vi "NI-DAQmxOLD.vi"() -> (0 "error out":errorcluster)   [LabVIEW 2022 SP3]
uses:
  Globals/Meas_global.vi
  <resource>/objmgr/daqmx.rc
  <vilib>/DAQmx/read.llb/DAQmx Read (Analog 2D DBL NChan NSamp).vi
  Sub_vis/Upload Data.ctl
  PWA/PWAtasksGLOBAL.vi
  <vilib>/DAQmx/create/channels.llb/DAQmx Create Channel (AI-Voltage-Basic).vi
  <vilib>/DAQmx/configure/timing.llb/DAQmx Timing (Sample Clock).vi
panel:
  out "FsReq":dbl
  out "FsRead":dbl format="%#_11g"
  out "input terminal configuration":i32(ring)=10106 items=["default"=-1, "RSE"=10083, "NRSE"=10078, "Differential"=10106, "Pseudodifferential"=12529]
  out "TotalSampPerChanAcquired":dbl=1024.0
  out "AvailSampPerChan":u32
  out "CurrReadPos":dbl=1024.0
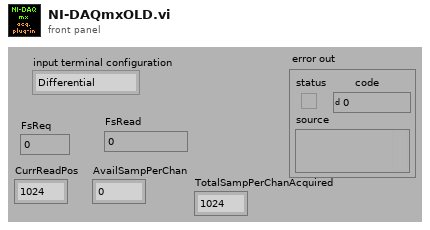
[diagram p1: front panel]
types:
  T1 = typedef "Analysis_info_cluster.ctl" = cluster{"Colour":u32, "Inst type":T2, "Inst name":string, "Symbol":string, "Code name":string, "Extra Info":string, "Inst Array":T3, "U":dbl, "u^2":dbl, "u^3":dbl, "u^4":dbl, "Skew_u":dbl, "Kurt_u":dbl, "Sd Error in Mean":dbl, "% u'/U":dbl, "X":dbl, "Y":dbl, "Z":dbl, "Timescale integral Estimate":dbl, "Sd Error in Variance":dbl, "Calib File":path, "Calib Constants":dbl[], "Output Position":bool, "Stats":enum16{"None", "Basic", "Full"}, "Av Sampling Rate":dbl, "Av No of Samples":dbl, "Total Meas Time (s)":dbl, "OrigChName":string, "Max value":dbl, "Min value":dbl, "Req Sample Rate Hz":dbl, "Sync Delay Time (s)":dbl, "Ch No":i16, "Device":string, "Use Latest Calib":bool, "Port":string, "Metadata Ch Names":string[], "Metadata Ch Values":string[], "Label":string, "chState":T4, "Point Drift":dbl, "inputConfig":string}
  T2 = typedef "Inst_type.ctl" = enum16{"Raw voltage", "Raw with zero offsetting", "Propeller anemometer", "Pressure Transducer", "Pitot-static tube", "Hot wire", "Cross wire 1", "Cross wire 2", "Generic Linear", "Generic Polynomial", "Generic BackPoly", "Fast FID", "Thermocouple", "Cold wire", "Pulsed Wire", "LDA Vel", "LDA Tran time", "LDA Arr time", "Microphone"}
  T3 = typedef "Instrument_Array.ctl" = enum16{"PWA", "LDA", "Analogue"}
  T4 = typedef "channelState.ctl" = enum32{"No Selection", "Solo", "Mute"}
  T5 = typedef "Device ID port info.ctl" = cluster{"Ch No":i16[], "Req Sampling Rate":dbl[], "Port":string, "Index":i32[]}
  T6 = typedef "Upload Data.ctl" = enum16{"Voltage Array", "Time Trace Cluster"}
  T7 = typedef "Setup.ctl" = enum16{"Run Program", "Show Setup", "Save Current Setup", "Setup Front Panel"}
  T8 = typedef "Rendezvous RefNum" = refnum<k1>
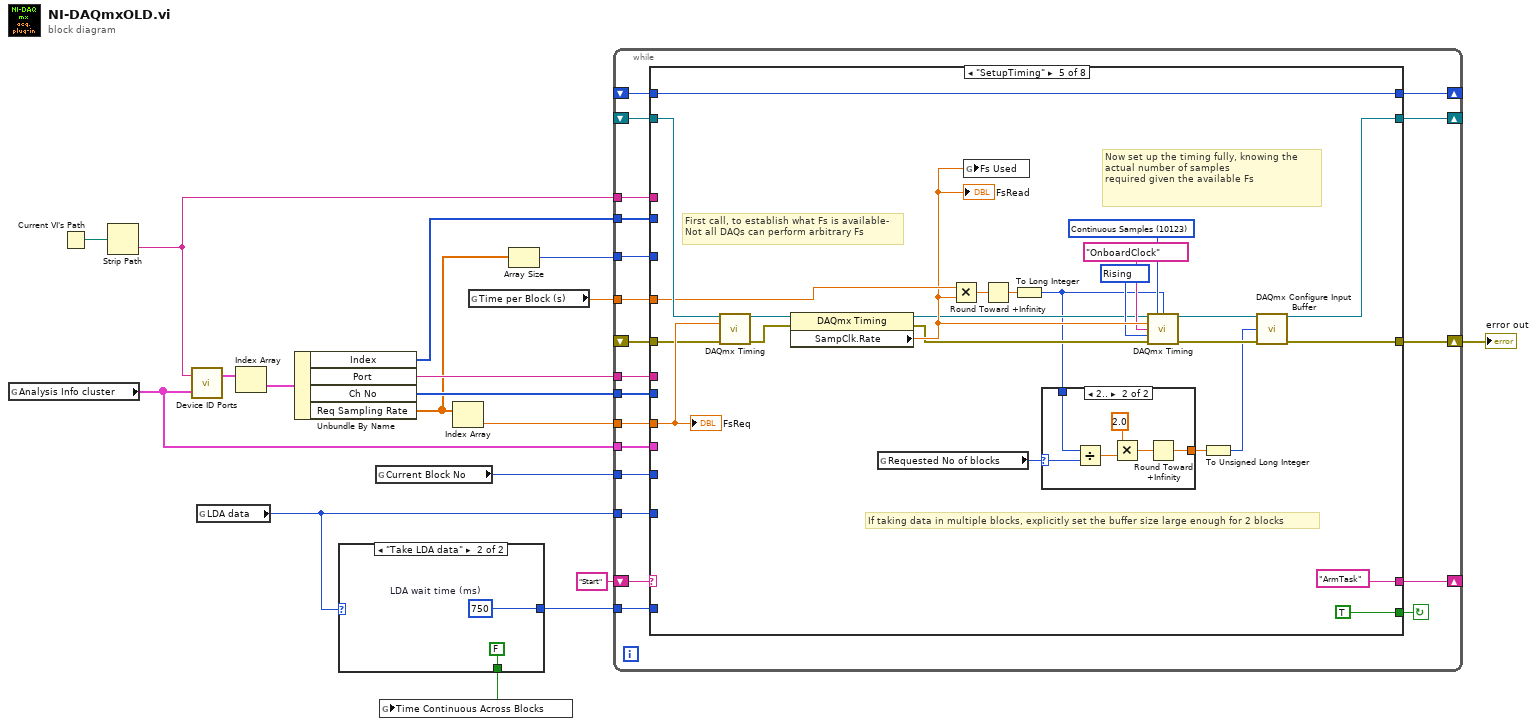
[diagram p0: block diagram]
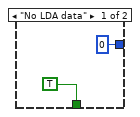
[diagram p2: hidden frame]
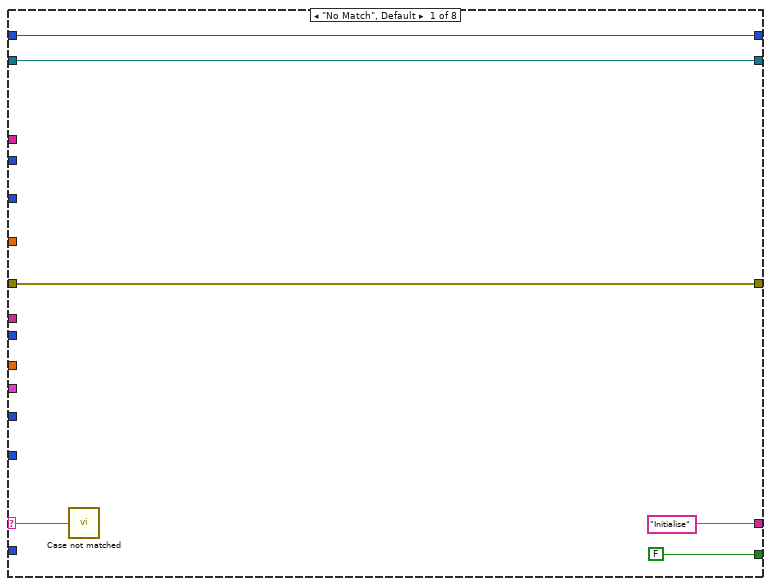
[diagram p3: hidden frame]
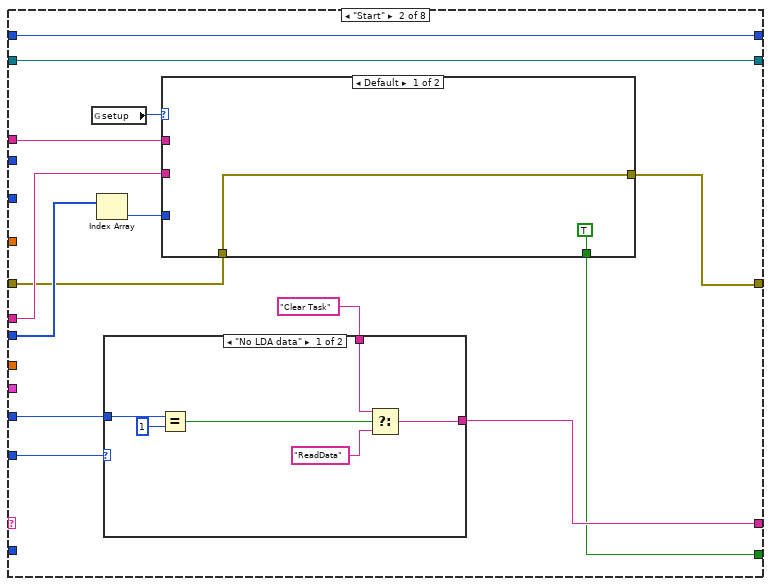
[diagram p4: hidden frame]
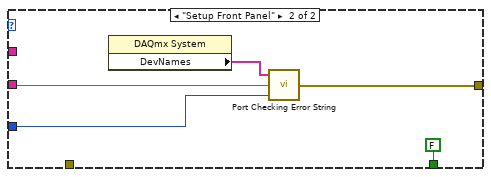
[diagram p5: hidden frame]
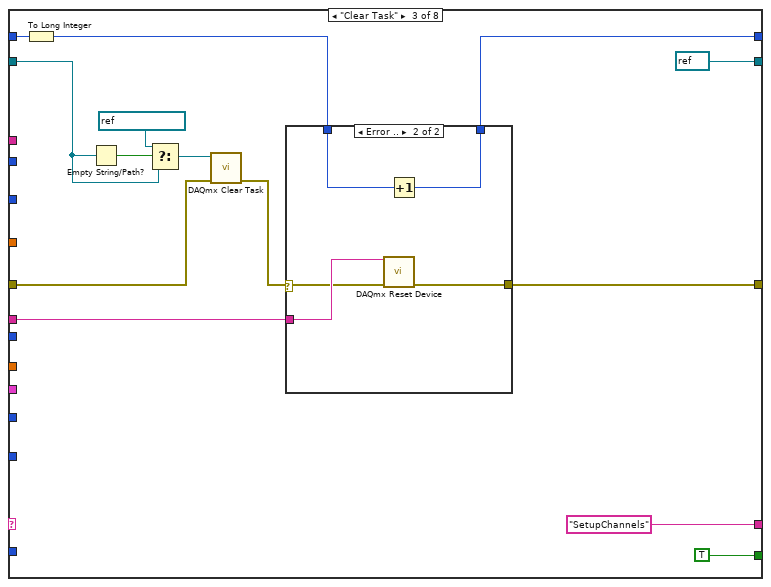
[diagram p7: hidden frame]
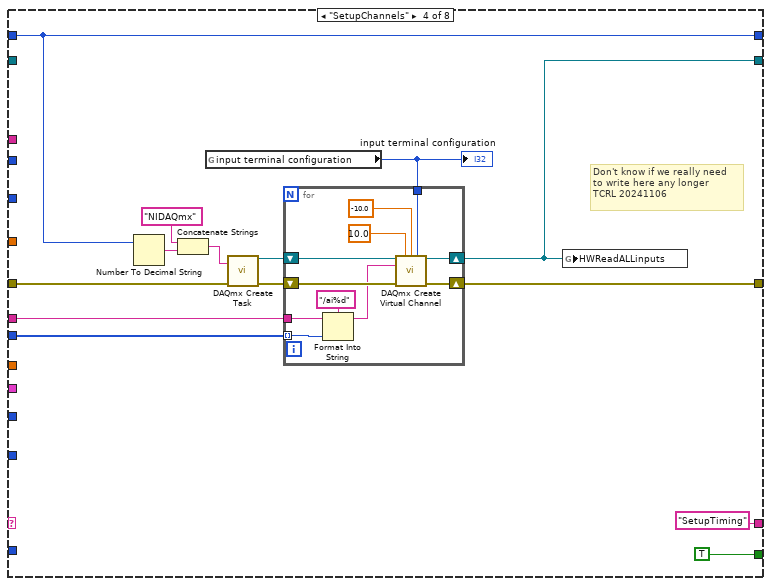
[diagram p9: hidden frame]
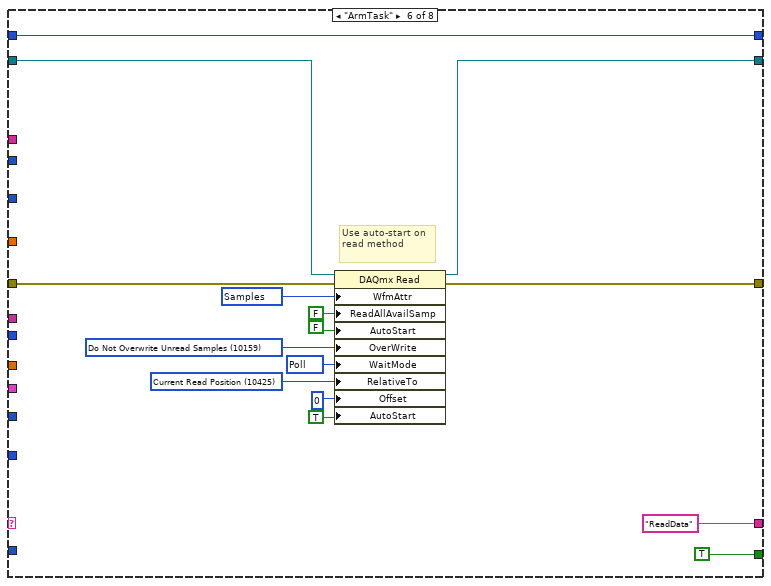
[diagram p11: hidden frame]
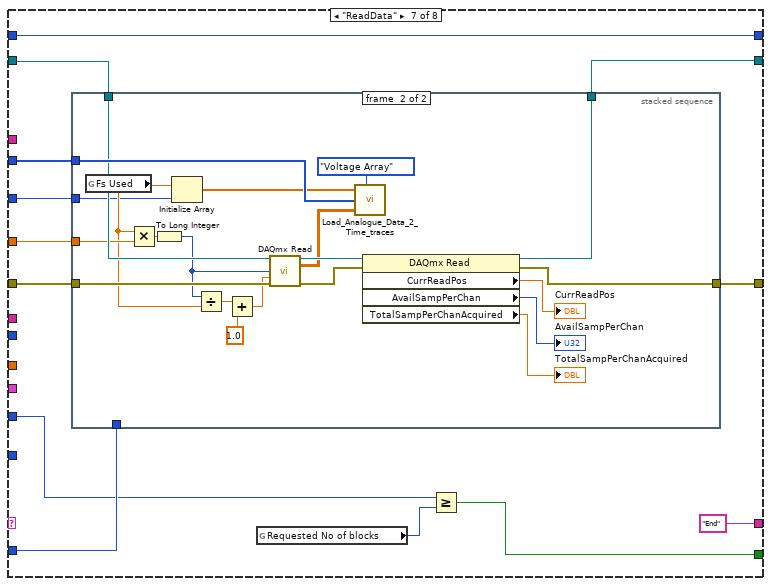
[diagram p12: hidden frame]
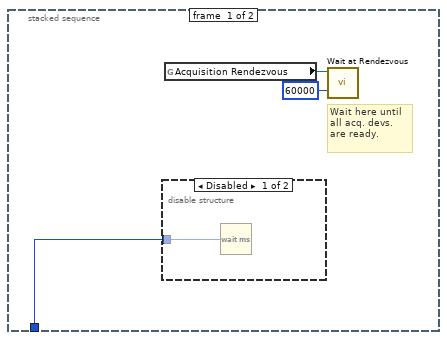
[diagram p13: hidden frame]
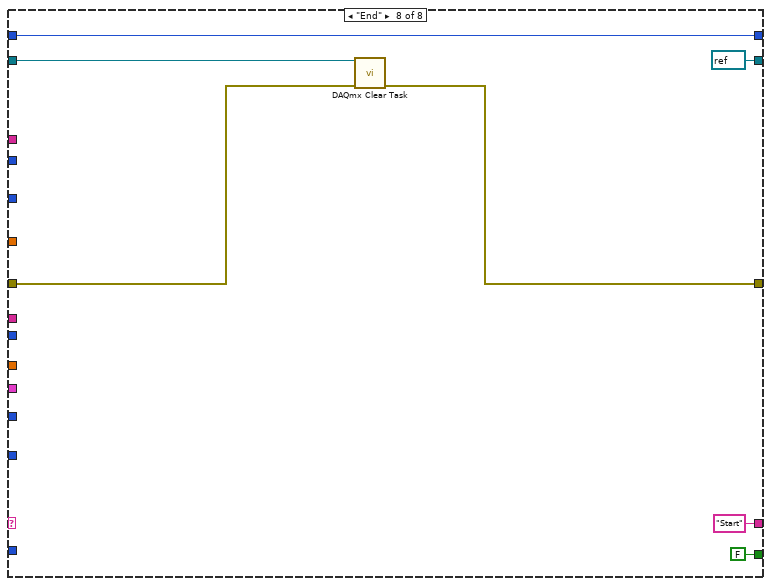
[diagram p15: hidden frame]
diagram:
  n1 = global read "Meas_global.vi" "Analysis Info cluster"() -> (w5:T1[])
  n2 = Current VI's Path() -> (path=w13:path)
  n3 = Strip Path(path=w13) -> (name=w6:string)  [unwired: 1 out]
  n4 = call "Device ID Ports.vi"("Analysis Info cluster"=w5, "DAQdeviceType"=w6) -> ("Device port info"=w11:T5[])  [unwired: 1 out]
  n5 = global read "Meas_global.vi" "LDA data"() -> (w17:enum16{"No LDA data", "Take LDA data"})
  n6 = Index Array(array=w11) -> (element=w10:T5)  [unwired: 1 in]
  n7 = Unbundle By Name(w10) -> ("Index"=w8:i32[], "Port"=w9:string, "Ch No"=w7:i16[], "Req Sampling Rate"=w1:dbl[])
  n8 = case shown="\"Take LDA data\"" w17 {
    tunnel: [TRUE ("Time Continuous across Blocks") FALSE ("Time Continuous across Blocks")] -> w16
    tunnel: [u32 0 ("LDA wait time (ms)") w21] -> w15
    frame "No LDA data" {
    }
    frame "Take LDA data" {
      w21 = u32 750  # LDA wait time (ms)
    }
  }
  n9 = global read "Meas_global.vi" "Current Block No"() -> (w3:i32)
  n10 = global write "Meas_global.vi" "Time Continuous Across Blocks"(w16) -> ()
  n11 = Index Array(array=w1) -> (element=w12:dbl)  [unwired: 1 in]
  n12 = global read "Meas_global.vi" "Time per Block (s)"() -> (w4:dbl)
  n13 = Array Size(array=w1) -> (size(s)=w2:i32)
  n14 = while {
    shift-left: "Start" -> [w42]
    shift-right: [w34] -> _
    shift-right: [w38] -> w14
    shift-left: _ -> [w41]
    tunnel: w12 -> [w40]
    tunnel: w3 -> [w39]
    shift-right: [w37] -> _
    shift-left: _ -> [w36]
    tunnel: w17 -> [w35]
    tunnel: w15 -> [w33]
    tunnel: w7 -> [w32]
    tunnel: w9 -> [w31]
    tunnel: w8 -> [w30]
    tunnel: w6 -> [w29]
    tunnel: w5 -> [w28]
    tunnel: w4 -> [w26]
    shift-right: [w25] -> _
    shift-left: _ -> [w24]
    tunnel: w2 -> [w23]
    stop <- w27 continue-if-true
    n15 = case shown="\"SetupTiming\"" w42 {
      selector: w42 -> [w43 _ _ _ _ _ _ _]
      tunnel: [FALSE w51 TRUE TRUE TRUE TRUE w172 FALSE] -> w27
      tunnel: ["Initialise" w61 "SetupChannels" "SetupTiming" "ArmTask" "ReadData" "End" "Start" ("f")] -> w34
      tunnel: [w46 w52 w84 w99 w127 w165 w177 w209] -> w38
      tunnel: w41 -> [w46 w49 w77 w100 w142 w168 w182 w208]
      tunnel: w40 -> [_ _ _ _ w144 _ _ _]
      tunnel: w39 -> [_ w59 _ _ _ _ w171 _]
      tunnel: [w45 w60 w82 w105 w145 w166 w180 w211] -> w37
      tunnel: w36 -> [w45 w60 w88 w105 w145 w166 w180 w211]
      tunnel: w35 -> [_ w58 _ _ _ _ _ _]
      tunnel: w33 -> [_ _ _ _ _ _ w179 _]
      tunnel: w32 -> [_ w54 _ w103 _ _ _ _]
      tunnel: w31 -> [_ w55 w86 w102 _ _ _ _]
      tunnel: w30 -> [_ _ _ _ _ _ w178 _]
      tunnel: w29 -> [_ w57 _ _ _ _ _ _]
      tunnel: w28 -> [_ _ _ _ _ _ _ _]
      tunnel: w26 -> [_ _ _ _ w141 _ w174 _]
      tunnel: [w44 w50 refnum<k21> refnum ("HWReadALLinputs") w98 w126 w163 w175 refnum<k21> refnum ("task out")] -> w25
      tunnel: w24 -> [w44 w50 w87 _ w143 w164 w176 w214]
      tunnel: w23 -> [_ _ _ _ _ _ w173 _]
      frame "No Match", Default {
        n16 = call "Case not matched.vi"("Case Name not Matched"=w43) -> ()
      }
      frame "Start" {
        n17 = global read "Meas_global.vi" "setup"() -> (w56:T7)
        n18 = Index Array(array=w54) -> (element=w53:i16)  [unwired: 1 in]
        n19 = case shown="\"No LDA data\"" w58 {
          tunnel: "Clear Task" -> [w75 w76]
          tunnel: [w73 w76] -> w61
          tunnel: w59 -> [w72 _]
          frame "No LDA data" {
            n20 = Equal?(x=w72, y=1) -> (x = y?=w70:bool)
            n21 = Select(t=w75, s=w70, f="ReadData") -> (s? t:f=w73:string)
          }
          frame "Take LDA data" {
          }
        }
        n22 = case shown="Default" w56 {
          tunnel: w57 -> [_ _]
          tunnel: w55 -> [_ w68]
          tunnel: w53 -> [_ w69]
          tunnel: [w63 w67] -> w52
          tunnel: [TRUE FALSE] -> w51
          tunnel: w49 -> [w63 _]
          frame Default {
          }
          frame "Setup Front Panel" {
            n23 = property class="DAQmx System"() -> ("DevNames"=w65:tag[])  [unwired: 2 in, 2 out]
            n24 = call "Port Checking Error String.vi"("Ch Index"=w69, "Port"=w68, "Available Ports"=w65) -> ("error out"=w67:errorcluster)  [unwired: 1 in]
          }
        }
      }
      frame "Clear Task" {
        n25 = To Long Integer(number=w88) -> (32bit integer=w83:i32)
        n26 = Empty String/Path?(string/path=w87) -> (empty?=w81:bool)
        n27 = Select(t=refnum<k21> "NIDAQmx0" ("HWReadALLinputs"), s=w81, f=w87) -> (s? t:f=w79:refnum<k21>)
        n28 = call <vilib>:"DAQmx Clear Task.vi"("task in"=w79, "error in"=w77) -> ("error out"=w78:errorcluster)  [unwired: 13 out]
        n29 = case shown="Error .." w78 {
          selector: w78 -> [w92 w93]
          tunnel: w86 -> [_ w97]
          tunnel: [w92 w96] -> w84
          tunnel: w83 -> [w91 w95]
          tunnel: [w91 w94] -> w82
          frame No Error {
          }
          frame Error {
            n30 = call <vilib>:"DAQmx Reset Device.vi"("device in"=w97, "error in"=w93) -> ("error out"=w96:errorcluster)  [unwired: 13 in]
            n31 = Increment(x=w95) -> (x+1=w94:i32)
          }
        }
      }
      frame "SetupChannels" {
        # "Don't know if we really need\nto write here any longer\nTCRL 20241106"
        n32 = Number To Decimal String(number=w105) -> (decimal integer string=w104:string)  [unwired: 1 in]
        n33 = Concatenate Strings("NIDAQmx" ("new task name"), w104) -> (w106:string)
        n34 = global read "Meas_global.vi" "input terminal configuration"() -> (w101:i32)
        "input terminal configuration" <- w101
        n35 = call <vilib>:"DAQmx Create Task.vi"("new task name"=w106, "error in"=w100) -> ("task out"=w109:refnum<k21>, "error out"=w110:errorcluster)  [unwired: 3 in, 9 out]
        n36 = for {
          shift-right: [w121] -> w98
          shift-left: w109 -> [w122]
          shift-right: [w119] -> w99
          shift-left: w110 -> [w120]
          tunnel: w103 -> [w116] mode=indexing
          tunnel: w102 -> [w115]
          tunnel: w101 -> [w112]
          n37 = Format Into String(format string="/ai%d", initial string=w115, w116) -> (resulting string=w117:string)  [unwired: 1 in, 1 out]
          n38 = call-poly <vilib>:"DAQmx Create Virtual Channel.vi"("task in"=w122, "maximum value"=10.0, "minimum value"=-10.0, "input terminal configuration"=w112, "physical channels"=w117, "error in"=w120) -> ("task out"=w121:refnum<k21>, "error out"=w119:errorcluster)  [unwired: 3 in, 5 out]
        }
        n39 = global write "PWAtasksGLOBAL.vi" "HWReadALLinputs"(w98) -> ()
      }
      frame "SetupTiming" {
        w135 = 10280 items=["Rising"=10280, "Falling"=10171] ("active edge")
        w138 = 10123 items=["Finite Samples"=10178, "Continuous Samples"=10123, "Hardware Timed Single Point"=12522] ("sample mode")
        # "If taking data in multiple blocks, explicitly set the buffer size large enough for 2 blocks"
        # "Now set up the timing fully, knowing the actual number of samples\nrequired given the available Fs"
        # "First call, to establish what Fs is available-\nNot all DAQs can perform arbitrary Fs"
        n40 = call-poly <vilib>:"DAQmx Timing.vi"("task/channels in"=w143, "rate"=w144, "error in"=w142) -> ("task out"=w140:refnum<k21>, "error out"=w133:errorcluster)  [unwired: 4 in, 7 out]
        n41 = property class="DAQmx Timing"(reference=w140, error in=w133) -> (reference out=w134:refnum<k21>, error out=w132:errorcluster, "SampClk.Rate"=w137:dbl)
        "FsRead" <- w137
        n42 = global read "Meas_global.vi" "Requested No of blocks"() -> (w125:i32)
        n43 = Multiply(x=w141, y=w137) -> (x*y=w139:dbl)
        n44 = global write "Meas_global.vi" "Fs Used"(w137) -> ()
        n45 = Round Toward +Infinity(x=w139) -> (ceil(x): smallest int >= x=w131:dbl)
        n46 = To Long Integer(number=w131) -> (32bit integer=w130:i32)
        n47 = case shown="2.." w125 {
          selector: w125 -> [_ w151]
          tunnel: w130 -> [w148 w152]
          tunnel: [w148 w150] -> w124
          frame 1, Default {
          }
          frame 2.. {
            n48 = Divide(x=w152, y=w151) -> (x/y=w154:dbl)
            n49 = Multiply(x=2.0, y=w154) -> (x*y=w149:dbl)
            n50 = Round Toward +Infinity(x=w149) -> (ceil(x): smallest int >= x=w150:dbl)
          }
        }
        n51 = call-poly <vilib>:"DAQmx Timing.vi"("task/channels in"=w134, "sample mode"=w138, "samples per channel"=w130, "rate"=w137, "source"=tag "OnboardClock", "active edge"=w135, "error in"=w132) -> ("task out"=w128:refnum<k21>, "error out"=w129:errorcluster)  [unwired: 7 out]
        n52 = To Unsigned Long Integer(number=w124) -> (unsigned 32bit integer=w123:u32)
        n53 = call <vilib>:"DAQmx Configure Input Buffer.vi"("task/channels in"=w128, "buffer size (in samples per channel)"=w123, "error in"=w129) -> ("task out"=w126:refnum<k21>, "error out"=w127:errorcluster)  [unwired: 11 in]
        "FsReq" <- w144
      }
      frame "ArmTask" {
        w157 = 10425 items=["First Sample"=10424, "Current Read Position"=10425, "Reference Trigger"=10426, "First Pretrigger Sample"=10427, "Most Recent Sample"=10428] ("RelativeTo")
        w158 = 12524 items=["Wait For Interrupt"=12523, "Poll"=12524, "Yield"=12525, "Sleep"=12547] ("WaitMode")
        w159 = 10159 items=["Overwrite Unread Samples"=10252, "Do Not Overwrite Unread Samples"=10159] ("OverWrite")
        w162 = 10287 items=["Samples"=10287, "Samples and Timing"=10140, "Samples, Timing, and Attributes"=10141] ("WfmAttr")
        # "Use auto-start on read method"
        n54 = property class="DAQmx Read"(reference=w164, error in=w168, "WfmAttr"=w162, "ReadAllAvailSamp"=FALSE, "AutoStart"=FALSE, "OverWrite"=w159, "WaitMode"=w158, "RelativeTo"=w157, "Offset"=0, "AutoStart"=TRUE) -> (reference out=w163:refnum<k21>, error out=w165:errorcluster)
      }
      frame "ReadData" {
        n55 = stacked-sequence {
          tunnel: w182 -> [_ w207]
          tunnel: [_ w201] -> w177
          tunnel: w179 -> [w185 _]
          tunnel: w178 -> [_ w199]
          tunnel: w176 -> [_ w196]
          tunnel: [_ w195] -> w175
          tunnel: w174 -> [_ w190]
          tunnel: w173 -> [_ w187]
          frame #0 {
            # "Wait here until all acq. devs. are ready."
            n56 = disable-structure shown="Disabled" {
              disable-tunnel: w185 -> [w186 _]
              frame Disabled {
                n57 = Wait (ms)(milliseconds to wait=w186) -> ()  [unwired: 1 out]
              }
              frame Enabled {
              }
            }
            n58 = global read "Meas_global.vi" "Acquisition Rendezvous"() -> (w184:T8)
            n59 = call <vilib>:"Wait at Rendezvous.vi"("ms timeout (-1)"=60000, "rendezvous"=w184) -> ()  [unwired: 3 in, 3 out]
          }
          frame #1 {
            n60 = global read "Meas_global.vi" "Fs Used"() -> (w189:dbl)
            n61 = Multiply(x=w189, y=w190) -> (x*y=w191:dbl)
            n62 = To Long Integer(number=w191) -> (32bit integer=w188:i32)
            n63 = Initialize Array(w189, w187) -> (w198:dbl[])
            n64 = Divide(x=w188, y=w189) -> (x/y=w204:dbl)
            n65 = Add(x=w204, y=1.0) -> (x+y=w202:dbl)
            n66 = call-poly <vilib>:"DAQmx Read.vi"("task/channels in"=w196, "number of samples per channel"=w188, "timeout"=w202, "error in"=w207) -> ("task out"=w206:refnum<k21>, "data"=w200:dbl[][], "error out"=w205:errorcluster)  [unwired: 9 out]
            n67 = call "Load_Analogue_Data_2_Time_traces.vi"("Sampling Rate (Hz)"=w198, "Mode"=Upload_Data."Voltage Array", "Index"=w199, "Voltage Array"=w200) -> ()  [unwired: 3 in]
            n68 = property class="DAQmx Read"(reference=w206, error in=w205) -> (reference out=w195:refnum<k21>, error out=w201:errorcluster, "CurrReadPos"=→"CurrReadPos":dbl, "AvailSampPerChan"=→"AvailSampPerChan":u32, "TotalSampPerChanAcquired"=→"TotalSampPerChanAcquired":dbl)
          }
        }
        n69 = global read "Meas_global.vi" "Requested No of blocks"() -> (w170:i32)
        n70 = Greater Or Equal?(x=w171, y=w170) -> (x >= y?=w172:bool)
      }
      frame "End" {
        n71 = call <vilib>:"DAQmx Clear Task.vi"("task in"=w214, "error in"=w208) -> ("error out"=w209:errorcluster)  [unwired: 13 out]
      }
    }
  }
  "error out" <- w14
